vi "Tag Engine Test 1.vi"() -> ()   [LabVIEW 2018]
uses:
  <vilib>/Utility/Data Type/Type Definitions/Data Type.ctl
  Tag/Tag.lvclass/Tag.ctl
  Core/Tag Core.lvclass/Tag Core.ctl
  d0cd855c-b644-45be-9fd4-ac58307db791.vi
  6bf29760-4029-4e6b-9ee1-3b5490a0454c.vi
  7d7e932f-16a3-47e4-8aaa-709ed214aa7d.vi
  363a3b3d-bf14-4d6f-8544-e87745e87888.vi
  a7708cd9-ec55-481d-a768-58ab3ae8be35.vi
  Tag/Construct.vi
  Tag/Write SetRequest.vi
  Core/Get Tag.vi
  7d7e932f-16a3-47e4-8aaa-709ed214aa7d.vi/b8b0363c-6996-44f6-a03d-aeec2e8f92c8.vi
  363a3b3d-bf14-4d6f-8544-e87745e87888.vi/bfa71975-dcc1-42d7-84c0-2d6dd5ef0689.vi
  Tag/Read Name.vi
  Tag/Read SetRequest Event.vi
  Tag/Read ValChange.vi
  a7708cd9-ec55-481d-a768-58ab3ae8be35.vi/3a8f494b-a0cc-4b43-b5b3-80dc6f810021.vi
  Tag/Write Value with Timestamp.vi
  Tag/Set Properties from Initial.vi
  Core/Add Tag.vi
  Core/Get Tag LUT.vi
  <vilib>/Utility/error.llb/Error Cluster From Error Code.vi
  Tag/Tag.lvclass
  Core/Tag Core.lvclass
  <vilib>/Utility/Data Type/NI_Data Type.lvlib
panel:
  out "Type":T1
  out "Tag Names":string[](array[string])
  out "error out":errorcluster
  out "New Time Stamp":timestamp
  out "New Value":variant
  out "Old Time Stamp":timestamp
  out "Old Value":variant
  out "Tag Name":string
  in  "stop":bool
  in  "Write":bool
  in  "Value":dbl
  in  "Name":string
  in  "Array":string[](array[string])=["{\"name\":\"Test1\",\"type\":\"Double Float\",\"description\":\"\",\"initial\":0,\"max\":Infinity,\"min\":-Infinity,\"default\":NaN,\"units\":\"\"}", "{\"name\":\"Test2\",\"type\":\"Double Float\",\"description\":\"\",\"initial\":0,\"max\":Infinity,\"min\":-Infinity,\"default\":NaN,\"units\":\"\"}"]
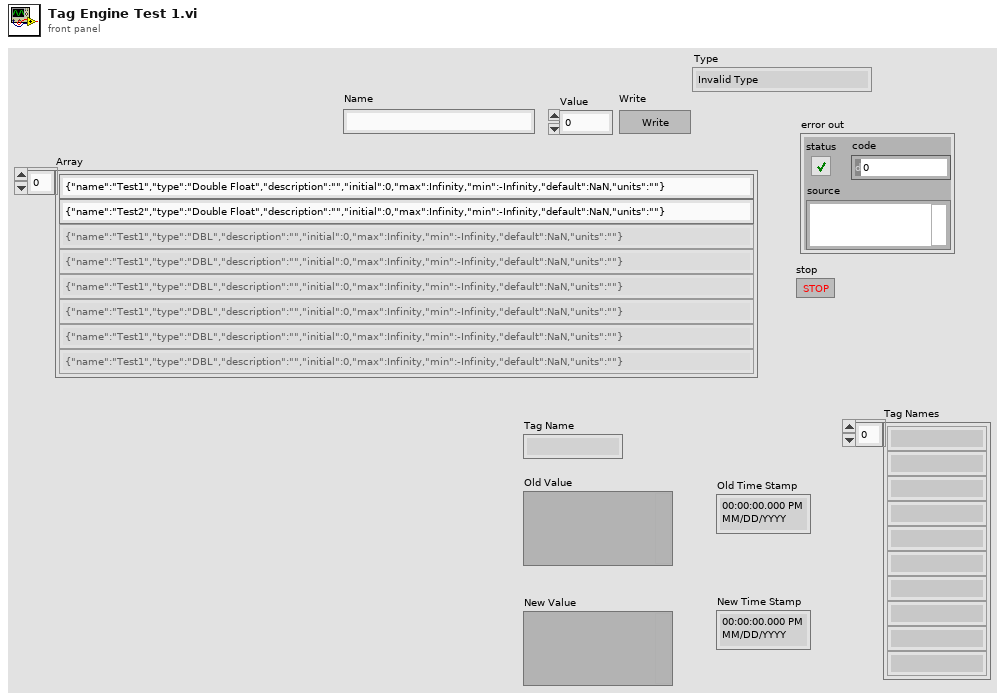
[diagram p1: front panel]
types:
  T1 = typedef "NI_Data Type.lvlib/Data Type.ctl" = enum8{"Invalid Type", "Void", "I8", "I16", "I32", "I64", "U8", "U16", "U32", "U64", "Single Float", "Double Float", "Extended Float", "Single Complex", "Double Complex", "Extended Complex", "Enum U8", "Enum U16", "Enum U32", "Enum U64", "Single Float With Unit", "Double Float With Unit", "Extended Float With Unit", "Single Complex with Unit", "Double Complex with Unit", "Extended Complex with Unit", "Boolean", "String", "Path", "Picture", "Tag", "Array", "Cluster", "Variant", "LV Variant", "Waveform", "Timestamp", "Digital Waveform", "Digital Data", "ExpressData", "Refnum", "External Data", "VI", "Poly VI", "LabVIEW Class Instance", "Fixed Point"}
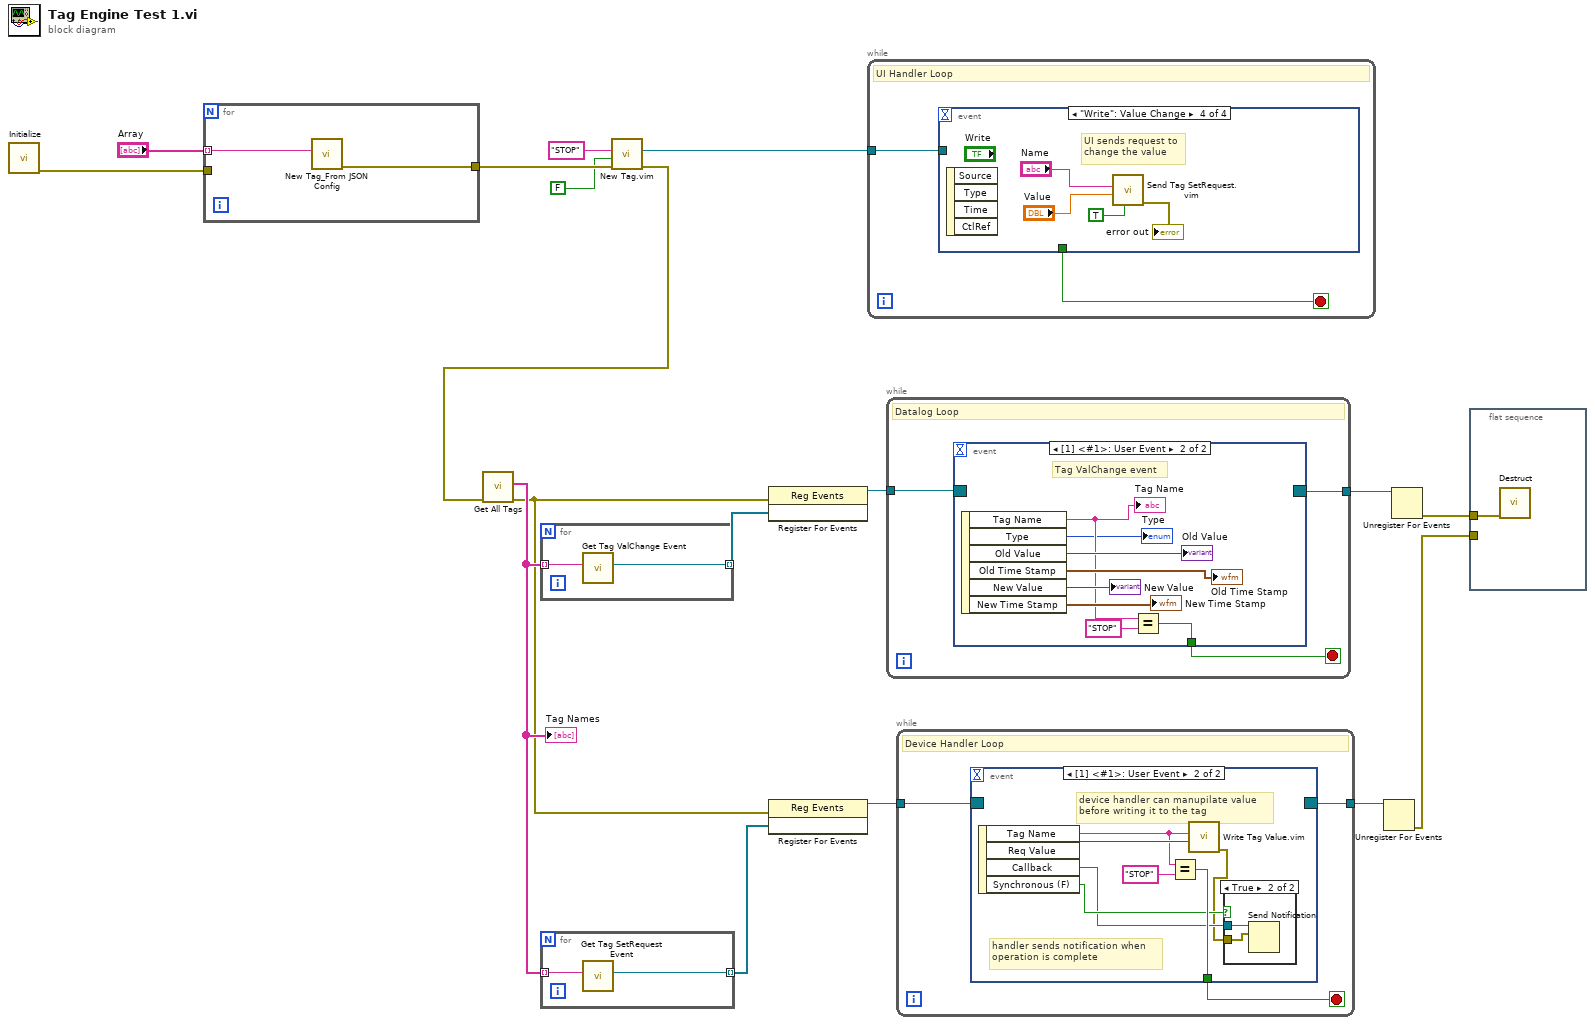
[diagram p0: block diagram]
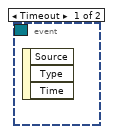
[diagram p2: hidden frame]
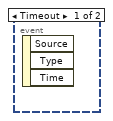
[diagram p4: hidden frame]
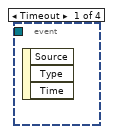
[diagram p5: hidden frame]
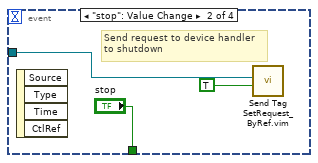
[diagram p6: hidden frame]
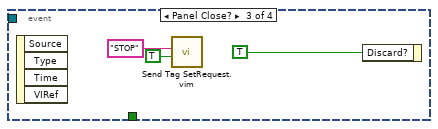
[diagram p7: hidden frame]
diagram:
  n1 = call "Initialize.vi"() -> ("error out"=w16:errorcluster)  [unwired: 11 in]
  n2 = for {
    tunnel: "Array" -> [w19] mode=indexing
    tunnel: w16 -> [_]
    tunnel: [w18] -> w11
    n3 = call "New Tag_From JSON Config.vi"("JSON Tag Config"=w19) -> ("error out"=w18:errorcluster)  [unwired: 9 in, 1 out]
  }
  n4 = call "New Tag.vim"("error in (no error)"=w11, "Initial Value"=FALSE, "Tag Name"="STOP" ("Name")) -> ("error out"=w10:errorcluster, "Tag Ref out"=w1:refnum<data-value>)  [unwired: 7 in]
  n5 = call "Get All Tags.vi"("error in (no error)"=w10) -> ("error out"=w2:errorcluster, "Tag Names"=w7:string[])  [unwired: 8 in, 1 out]
  "Tag Names" <- w7
  n6 = for {
    tunnel: w7 -> [w21] mode=indexing
    tunnel: [w20] -> w13 mode=indexing
    n7 = call "Get Tag ValChange Event.vi"("Tag Name"=w21) -> ("ValChange"=w20:refnum<user-event>)  [unwired: 9 in, 1 out]
  }
  n8 = for {
    tunnel: w7 -> [w23] mode=indexing
    tunnel: [w22] -> w6 mode=indexing
    n9 = call "Get Tag SetRequest Event.vi"("Tag Name"=w23) -> ("SetRequest"=w22:refnum<user-event>)  [unwired: 9 in, 1 out]
  }
  n10 = register-events(error in=w2, w13) -> (reference out=w12:refnum<event-registration>)  [unwired: 1 in, 1 out]
  n11 = register-events(error in=w2, w6) -> (reference out=w5:refnum<event-registration>)  [unwired: 1 in, 1 out]
  n12 = while {
    tunnel: w1 -> [w24]
    stop <- w25 stop-if-true
    # "UI Handler Loop"
    n13 = event shown="[3] \"Write\": Value Change" {
      selector: _ -> [_ _ _ _]
      dyn-events: _ -> [_ _ _ _]
      timeout: _ -> [_ _ _ _]
      tunnel: [_ "stop" _ _] -> w25
      tunnel: w24 -> [_ w27 _ _]
      event Timeout {
        n14 = event-data() -> ()  [unwired: 1 in, 3 out]
      }
      event "stop": Value Change {
        # "Send request to device handler\nto shutdown"
        n15 = event-data() -> ()  [unwired: 1 in, 4 out]
        n16 = call "Send Tag SetRequest_ByRef.vim"("Value"=TRUE, "Tag Ref in"=w27) -> ()  [unwired: 7 in, 3 out]
      }
      event Panel Close? {
        n17 = event-data() -> ()  [unwired: 1 in, 4 out]
        n18 = call "Send Tag SetRequest.vim"("Value"=TRUE, "Tag Name(s)/Ref(s)"="STOP" ("Name")) -> ()  [unwired: 8 in, 2 out]
        n19 = event-data("Discard?"=TRUE) -> ()  [unwired: 1 in, 1 out]
      }
      event "Write": Value Change {
        # "UI sends request to\nchange the value"
        n20 = event-data() -> ()  [unwired: 1 in, 4 out]
        n21 = call "Send Tag SetRequest.vim"("Synchronous (F)"=TRUE, "Value"="Value", "Tag Name(s)/Ref(s)"="Name") -> ("error out"=→"error out":errorcluster)  [unwired: 7 in, 1 out]
      }
    }
  }
  n22 = while {
    tunnel: [w38] -> w15
    tunnel: w12 -> [w37]
    stop <- w36 stop-if-true
    # "Datalog Loop"
    n23 = event shown="[1] <#1>: User Event" {
      selector: w37 -> [_ _]
      dyn-events: [_ _] -> w38
      timeout: _ -> [_ _]
      tunnel: [_ w40] -> w36
      event Timeout {
        n24 = event-data() -> ()  [unwired: 1 in, 3 out]
      }
      event User Event {
        # "Tag ValChange event"
        n25 = event-data() -> ("Tag Name"=w42:string, "Type"=→"Type":T1, "Old Value"=→"Old Value":variant, "Old Time Stamp"=→"Old Time Stamp":timestamp, "New Value"=→"New Value":variant, "New Time Stamp"=→"New Time Stamp":timestamp)  [unwired: 1 in]
        "Tag Name" <- w42
        n26 = Equal?(x=w42, y="STOP") -> (x = y?=w40:bool)
      }
    }
  }
  n27 = while {
    tunnel: w5 -> [w49]
    tunnel: [w47] -> w4
    stop <- w48 stop-if-true
    # "Device Handler Loop"
    n28 = event shown="[1] <#1>: User Event" {
      selector: w49 -> [_ _]
      dyn-events: [_ _] -> w47
      timeout: _ -> [_ _]
      tunnel: [_ w53] -> w48
      event Timeout {
        n29 = event-data() -> ()  [unwired: 1 in, 3 out]
      }
      event User Event {
        # "handler sends notification when\noperation is complete"
        # "device handler can manupilate value\nbefore writing it to the tag"
        n30 = event-data() -> ("Tag Name"=w55:string, "Req Value"=w56:variant, "Callback"=w51:refnum<notifier>, "Synchronous (F)"=w52:bool)  [unwired: 1 in]
        n31 = Equal?(x=w55, y="STOP") -> (x = y?=w53:bool)
        n32 = call "Write Tag Value.vim"("Value"=w56, "Tag Name(s)/Ref(s)"=w55) -> ("error out"=w50:errorcluster)  [unwired: 8 in, 1 out]
        n33 = case shown="True" w52 {
          tunnel: w51 -> [_ w58]
          tunnel: w50 -> [_ w57]
          frame False {
          }
          frame True {
            n34 = Send Notification(notification=w57, notifier=w58) -> ()  [unwired: 1 in, 2 out]
          }
        }
      }
    }
  }
  n35 = Unregister For Events(event registration refnum=w4) -> (error out=w3:errorcluster)  [unwired: 1 in]
  n36 = Unregister For Events(event registration refnum=w15) -> (error out=w14:errorcluster)  [unwired: 1 in]
  n37 = flat-sequence {
    tunnel: w14 -> [w59]
    tunnel: w3 -> [_]
    frame #0 {
      n38 = call "Destruct.vi"("error in (no error)"=w59) -> ()  [unwired: 10 in, 1 out]
    }
  }
